vi "ServoPWMGenerator.vi"(4 "ZeroLatch":bool[](array[boolean])=[FALSE, FALSE, FALSE, FALSE, FALSE, FALSE, FALSE, FALSE, FALSE, FALSE], 5 "Enabled":bool, 6 "MinHigh":u16, 7 "Period":u16, 8 "PeriodScale":u8[](array[numeric])=[0, 0, 0, 0, 0, 0, 0, 0, 0, 0], 9 "Inputs":u16[](array[numeric])=[0, 0, 0, 0, 0, 0, 0, 0, 0, 0]) -> (1 "Outputs":bool[](array[boolean]), 3 "PeriodStarted":bool)   [LabVIEW 2019]
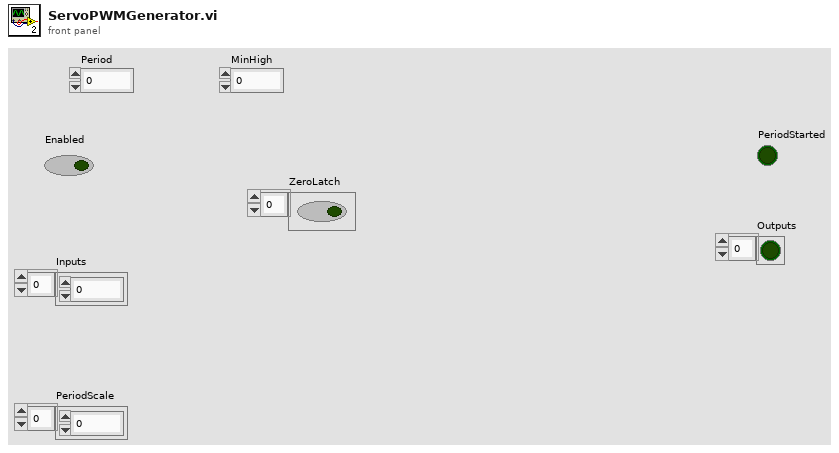
[diagram p1: front panel]
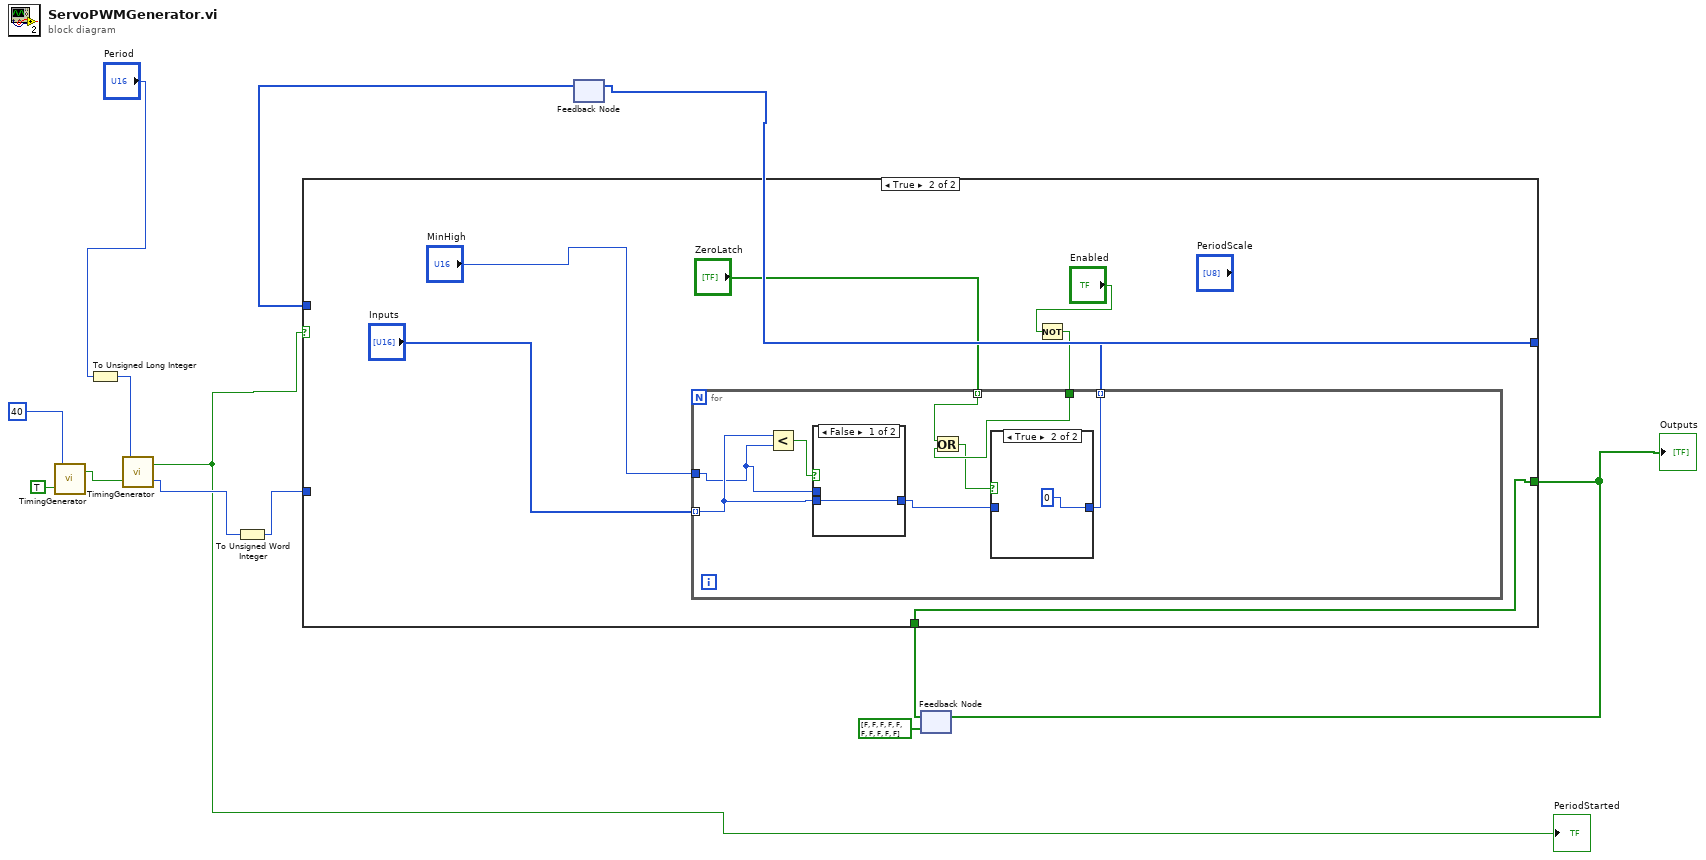
[diagram p0: block diagram]
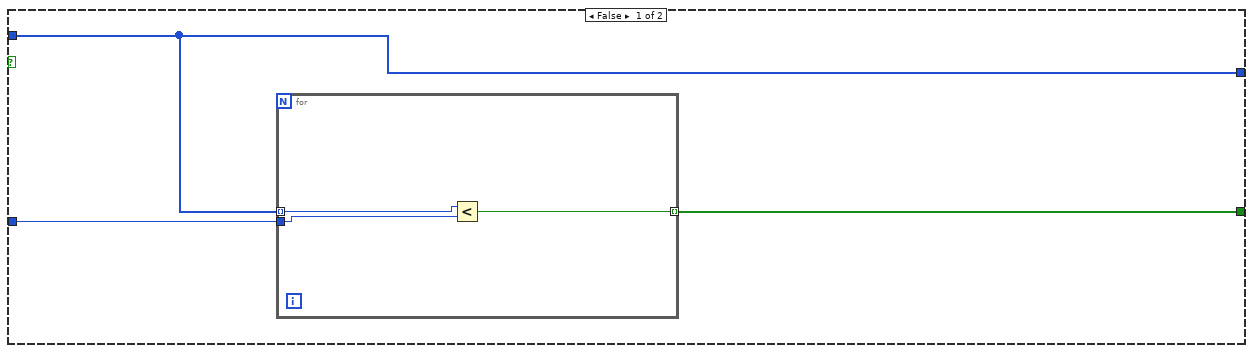
[diagram p2: hidden frame]
diagram:
  n1 = call "TimingGenerator.vi"("Tick"=TRUE, "Period"=u32 40 ("y")) -> ("Pulse"=w9:bool)  [unwired: 1 out]
  n2 = To Unsigned Long Integer(number="Period") -> (unsigned 32bit integer=w8:u32)
  n3 = call "TimingGenerator.vi"("Tick"=w9, "Period"=w8) -> ("TimeSinceLastPulse"=w4:u32, "Pulse"=w2:bool)
  "PeriodStarted" <- w2
  n4 = To Unsigned Word Integer(number=w4) -> (unsigned 16bit integer=w3:u16)
  n5 = feedback #1() -> (w12:u16[])  [unwired: 1 in]
  n6 = feedback #2(bool[] [FALSE, FALSE, FALSE, FALSE, FALSE, FALSE, FALSE, FALSE, FALSE, FALSE]) -> (w5:bool[])
  n7 = case shown="True" w2 {
    tunnel: [w16 w23] -> w13
    tunnel: w12 -> [w16 _]
    tunnel: w3 -> [w15 _]
    tunnel: [w14 w22] -> w6
    tunnel: w5 -> [_ w22]
    frame False {
      n8 = for {
        tunnel: w16 -> [w19] mode=indexing
        tunnel: w15 -> [w18]
        tunnel: [w17] -> w14 mode=indexing
        n9 = Less?(x=w19, y=w18) -> (x < y?=w17:bool)
      }
    }
    frame True {
      n10 = Not(x="Enabled") -> (.not. x?=w20:bool)
      n11 = for {
        tunnel: "Inputs" -> [w33] mode=indexing
        tunnel: "MinHigh" -> [w32]
        tunnel: "ZeroLatch" -> [w29] mode=indexing
        tunnel: [w30] -> w23 mode=indexing
        tunnel: w20 -> [w28]
        n12 = Less?(x=w33, y=w32) -> (x < y?=w34:bool)
        n13 = case shown="False" w34 {
          tunnel: w33 -> [w37 _]
          tunnel: [w37 w38] -> w31
          tunnel: w32 -> [_ w38]
          frame False {
          }
          frame True {
          }
        }
        n14 = Or(x=w29, y=w28) -> (x .or. y?=w27:bool)
        n15 = case shown="True" w27 {
          tunnel: [w35 u16 0] -> w30
          tunnel: w31 -> [w35 _]
          frame False {
          }
          frame True {
          }
        }
      }
    }
  }
  "Outputs" <- w6
  n16 = feedback-in #1(w13) -> ()
  n17 = feedback-in #2(w6) -> ()
